vi "PDHydra -PWM Analysis.vi"(0 "Analysis Leg":i32, 5 "Active Leg":i32, 7 "Duty Cycle":i32=25, 9 "Waveform":waveform(dbl)[](array[waveform]), 11 "Board Selector":T1) -> (10 "Result (Boolean)":bool, 15 "Message":string)   [LabVIEW 2022 SP3]
uses:
  Serial Board Com/Board Select.ctl
  <vilib>/measure/mascope.llb/Pulse Measurements 1 chan.vi
  <vilib>/measure/madcrms.llb/Basic Averaged DC-RMS for 1 Chan.vi
  <vilib>/measure/NI_MAPro.lvlib
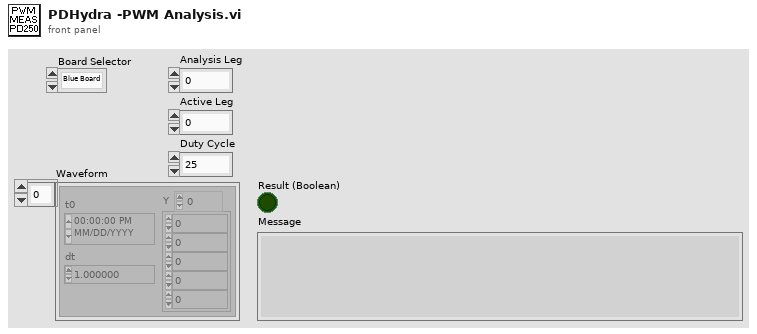
[diagram p1: front panel]
types:
  T1 = typedef "Board Select.ctl" = enum16{"Blue Board", "Green Board"}
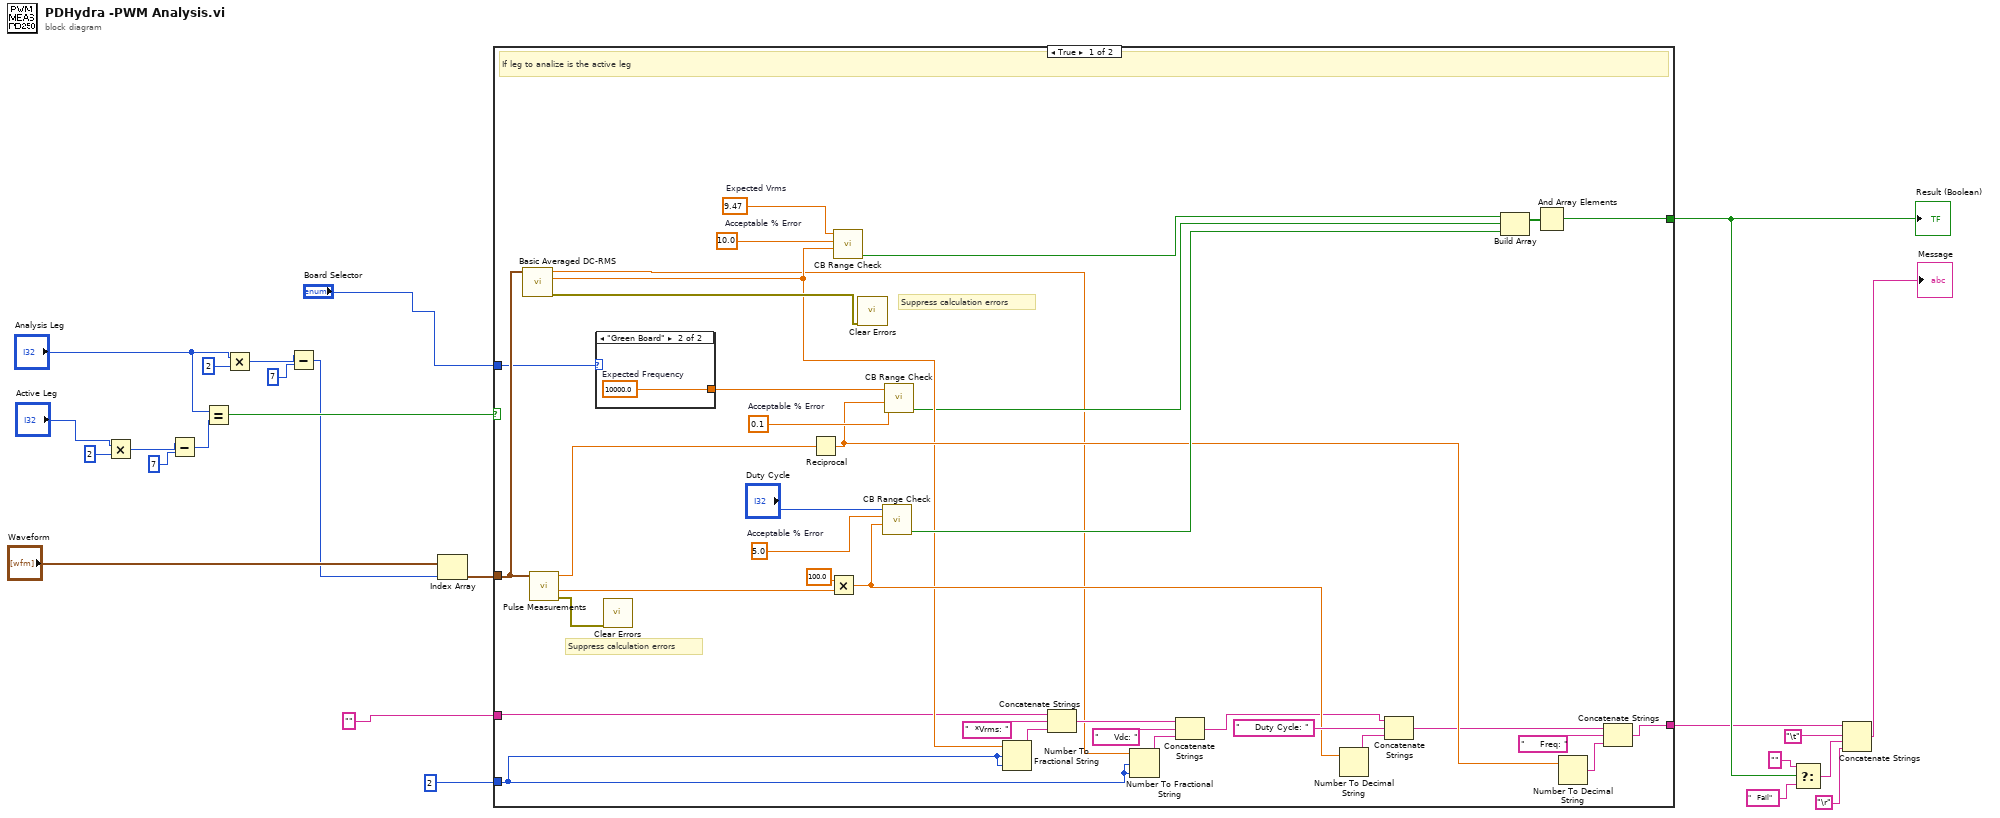
[diagram p0: block diagram]
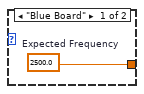
[diagram p2: hidden frame]
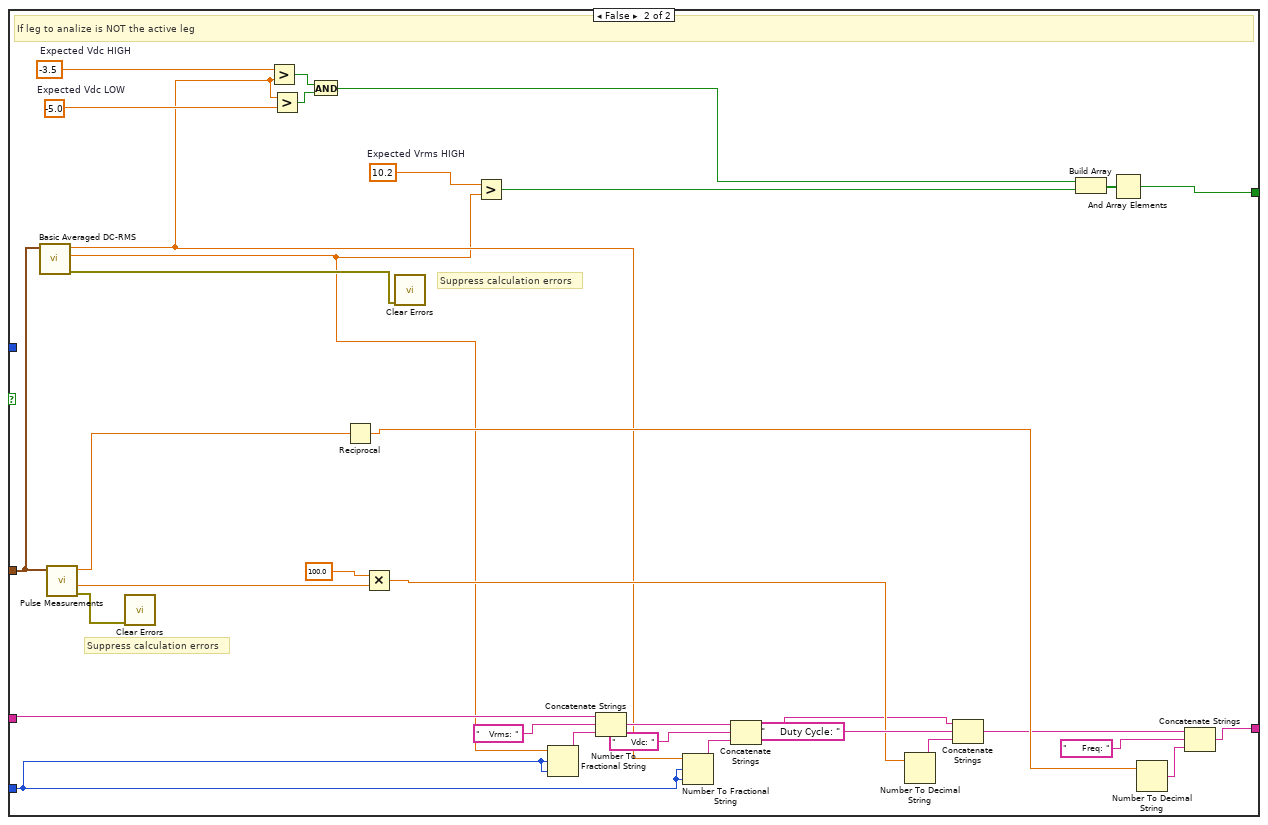
[diagram p3: hidden frame]
diagram:
  n1 = Multiply(x="Active Leg", y=2) -> (x*y=w4:i32)
  n2 = Subtract(x=w4, y=7) -> (x-y=w1:i32)
  n3 = Equal?(x="Analysis Leg", y=w1) -> (x = y?=w15:bool)
  n4 = Multiply(x="Analysis Leg", y=2) -> (x*y=w8:i32)
  n5 = Subtract(x=w8, y=7) -> (x-y=w6:i32)
  n6 = Index Array(array="Waveform", index=w6) -> (element=w21:waveform(dbl))
  n7 = case shown="True" w15 {
    tunnel: w21 -> [w45 w83]
    tunnel: [w39 w80] -> w17
    tunnel: [w28 w67] -> w16
    tunnel: "" -> [w30 w69]
    tunnel: 2 -> [w27 w66]
    tunnel: "Board Selector" -> [w25 _]
    frame True {
      w33 = 10.0  # Acceptable % Error
      w32 = 9.47  # Expected Vrms
      w53 = 5.0  # Acceptable % Error
      w54 = 0.1  # Acceptable % Error
      # "Suppress calculation errors"
      # "Suppress calculation errors"
      # "If leg to analize is the active leg"
      n8 = call-poly <vilib>:"Basic Averaged DC-RMS.vi"("signal in"=w45) -> ("error out"=w46:errorcluster, "RMS value"=w41:dbl, "DC value"=w31:dbl)  [unwired: 7 in, 1 out]
      n9 = call-poly <vilib>:"Pulse Measurements.vi"("signal in"=w45) -> ("error out"=w55:errorcluster, "duty cycle"=w57:dbl, "period"=w56:dbl)  [unwired: 6 in, 2 out]
      n10 = case shown="\"Green Board\"" w25 {
        tunnel: [w61 w62] -> w26
        frame "Blue Board" {
          w61 = 2500.0  # Expected Frequency
        }
        frame "Green Board" {
          w62 = 10000.0  # Expected Frequency
        }
      }
      n11 = call <vilib>:"Clear Errors.vi"("error in (no error)"=w55) -> ()  [unwired: 5 in, 2 out]
      n12 = Reciprocal(x=w56) -> (1/x=w47:dbl)
      n13 = Multiply(x=100.0, y=w57) -> (x*y=w50:dbl)
      n14 = call "CB Range Check.vi"("Actual Value"=w41, "Acceptable% Error"=w33, "Expected Value"=w32) -> ("Result (Boolean)"=w44:bool)  [unwired: 6 in, 2 out]
      n15 = call <vilib>:"Clear Errors.vi"("error in (no error)"=w46) -> ()  [unwired: 5 in, 2 out]
      n16 = call "CB Range Check.vi"("Actual Value"=w50, "Acceptable% Error"=w53, "Expected Value"="Duty Cycle") -> ("Result (Boolean)"=w58:bool)  [unwired: 6 in, 2 out]
      n17 = call "CB Range Check.vi"("Actual Value"=w47, "Acceptable% Error"=w54, "Expected Value"=w26) -> ("Result (Boolean)"=w40:bool)  [unwired: 6 in, 2 out]
      n18 = Number To Fractional String(number=w41, width (-)=w27, precision (6)=w27) -> (F-format string=w43:string)  [unwired: 1 in]
      n19 = Concatenate Strings(w30, "  *Vrms: " ("string"), w43) -> (w35:string)
      n20 = Number To Fractional String(number=w31, width (-)=w27, precision (6)=w27) -> (F-format string=w37:string)  [unwired: 1 in]
      n21 = Concatenate Strings(w35, "     Vdc: " ("string"), w37) -> (w29:string)
      n22 = Number To Decimal String(number=w50) -> (decimal integer string=w51:string)  [unwired: 1 in]
      n23 = Concatenate Strings(w29, "     Duty Cycle: " ("string"), w51) -> (w36:string)
      n24 = Build Array(w44, w40, w58) -> (w59:bool[])
      n25 = And Array Elements(Boolean array=w59) -> (logical AND=w39:bool)
      n26 = Number To Decimal String(number=w47) -> (decimal integer string=w48:string)  [unwired: 1 in]
      n27 = Concatenate Strings(w36, "     Freq: " ("string"), w48) -> (w28:string)
    }
    frame False {
      w65 = 10.2  # Expected Vrms HIGH
      w74 = -5.0  # Expected Vdc LOW
      w75 = -3.5  # Expected Vdc HIGH
      # "Suppress calculation errors"
      # "Suppress calculation errors"
      # "If leg to analize is NOT the active leg"
      n28 = call-poly <vilib>:"Basic Averaged DC-RMS.vi"("signal in"=w83) -> ("error out"=w84:errorcluster, "RMS value"=w64:dbl, "DC value"=w70:dbl)  [unwired: 7 in, 1 out]
      n29 = call-poly <vilib>:"Pulse Measurements.vi"("signal in"=w83) -> ("error out"=w91:errorcluster, "duty cycle"=w93:dbl, "period"=w92:dbl)  [unwired: 6 in, 2 out]
      n30 = call <vilib>:"Clear Errors.vi"("error in (no error)"=w91) -> ()  [unwired: 5 in, 2 out]
      n31 = Greater?(x=w75, y=w70) -> (0:w73:bool)
      n32 = Greater?(x=w70, y=w74) -> (0:w72:bool)
      n33 = And(x=w73, y=w72) -> (x .and. y?=w71:bool)
      n34 = Reciprocal(x=w92) -> (1/x=w85:dbl)
      n35 = Multiply(x=100.0, y=w93) -> (x*y=w88:dbl)
      n36 = call <vilib>:"Clear Errors.vi"("error in (no error)"=w84) -> ()  [unwired: 5 in, 2 out]
      n37 = Greater?(x=w65, y=w64) -> (0:w63:bool)
      n38 = Number To Fractional String(number=w64, width (-)=w66, precision (6)=w66) -> (F-format string=w82:string)  [unwired: 1 in]
      n39 = Concatenate Strings(w69, "   Vrms: " ("string"), w82) -> (w76:string)
      n40 = Number To Fractional String(number=w70, width (-)=w66, precision (6)=w66) -> (F-format string=w78:string)  [unwired: 1 in]
      n41 = Concatenate Strings(w76, "     Vdc: " ("string"), w78) -> (w68:string)
      n42 = Number To Decimal String(number=w88) -> (decimal integer string=w89:string)  [unwired: 1 in]
      n43 = Concatenate Strings(w68, "     Duty Cycle: " ("string"), w89) -> (w77:string)
      n44 = Build Array(w71, w63) -> (w94:bool[])
      n45 = And Array Elements(Boolean array=w94) -> (logical AND=w80:bool)
      n46 = Number To Decimal String(number=w85) -> (decimal integer string=w86:string)  [unwired: 1 in]
      n47 = Concatenate Strings(w77, "     Freq: " ("string"), w86) -> (w67:string)
    }
  }
  "Result (Boolean)" <- w17
  n48 = Select(t="" ("string"), s=w17, f="   Fail" ("string")) -> (s? t:f=w18:string)
  n49 = Concatenate Strings(w16, "\t", w18, "\r") -> (→"Message":string)
